vi "Read Pin.vi"(0 "Simulated Device in":refnum<class "Simulated Device.lvclass">, 5 "VISA resource name":refnum<visa-resource-name>, 9 "Port":dbl, 11 "error in (no error)":errorcluster) -> (4 "Simulated Device out":refnum<class "Simulated Device.lvclass">, 6 "VISA resource name 2":refnum<visa-resource-name>, 8 "Pin":bool, 10 "Response":string, 15 "error out":errorcluster)   [LabVIEW 2020, in "Simulated Device.lvclass"]
uses:
  Simulated Device.lvclass
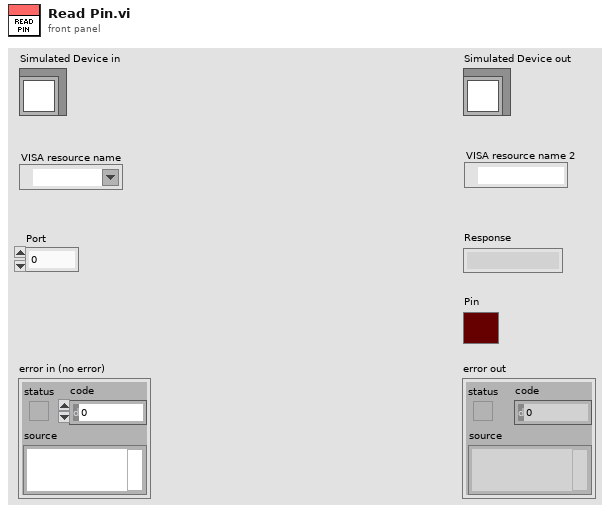
[diagram p1: front panel]
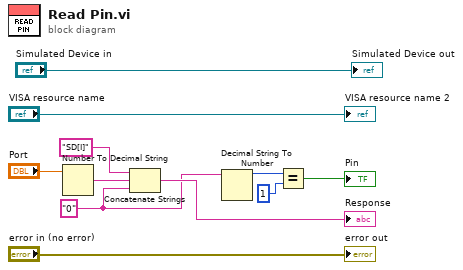
[diagram p0: block diagram]
diagram:
  w2 = "0" ("string")
  n1 = Number To Decimal String(number="Port") -> (decimal integer string=w7:string)  [unwired: 1 in]
  n2 = Concatenate Strings("SD[I]" ("string"), w7, w2) -> (→"Response":string)
  n3 = Decimal String To Number(string=w2) -> (offset past number=w5:i32)  [unwired: 2 in, 1 out]
  n4 = Equal?(x=w5, y=1) -> (x = y?=→"Pin":bool)
  "error out" <- "error in (no error)"
  "Simulated Device out" <- "Simulated Device in"
  "VISA resource name 2" <- "VISA resource name"
